vi "Test PA on multiple channels.vi"(11 "Test Case In":refnum<class "NI9375 DI Cont CFG.lvclass">) -> (0 "error out":errorcluster, 3 "Test Case Out":refnum<class "NI9375 DI Cont CFG.lvclass">)   [LabVIEW 2024, in "NI9375 DI Cont CFG.lvclass"]
uses:
  NI9375 DI Cont CFG.lvclass
  NI9375 DI Cont CFG.lvclass/NI9375 DI Cont CFG.ctl
  HAL/MSS/MSS.lvclass
  <vilib>/Astemes/LUnit/Test Case.lvclass
  <vilib>/platform/TimedLoop/XDataNode/XDataNode.xnode
  <vilib>/Platform/TimedLoop/XDataNode/nitl_modes.ctl
  <vilib>/Platform/TimedLoop/XDataNode/XDNodeRunTimeDep.lvlib
  <vilib>/Platform/TimedLoop/XDataNode/wakeup.ctl
  <vilib>/Platform/TimedLoop/XDataNode/timing_clust.ctl
panel:
  out "Error":errorcluster
  in  "stop":bool
  out "Output":variant
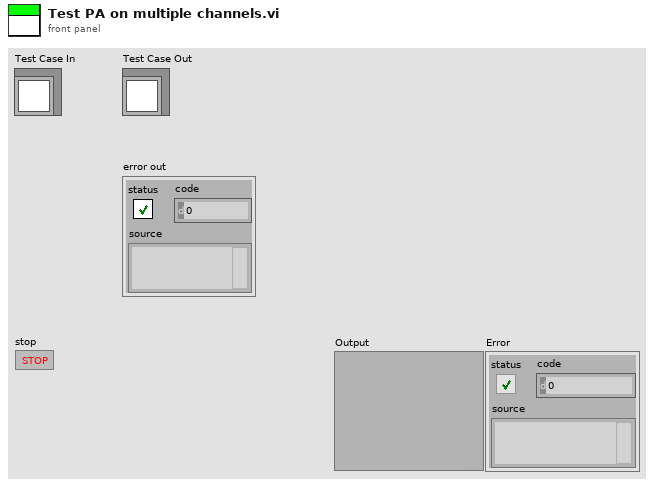
[diagram p1: front panel]
types:
  T1 = typedef "XDNodeRunTimeDep.lvlib/timing_clust.ctl" = cluster{"Expected End [f-1]":u64, "Actual End [f-1]":u64, "Finished Late? [f-1]":bool, "Expected End [i-1]":u64, "Actual End [i-1]":u64, "Finished Late? [i-1]":bool, "Expected Start [i]":u64, "Actual Start [i]":u64, "Expected Start [f]":u64, "Actual Start [f]":u64, "Source Name":string, "Structure Name":string, "Period":i64, "Deadline":i64, "Offset":i64, "Start":i64, "Priority":i32, "Timeout":i32, "Mode":T2, "Wakeup Reason":T3, "Error":errorcluster, "Source Type":string, "Secondary Source Type":string, "Global End Time":u64, "Global Start Time":u64, "Frame Duration":u64, "Iteration Duration":u64, "Assigned CPU":i32, "I/O Scan Engine Mode":u32}
  T2 = typedef "XDNodeRunTimeDep.lvlib/nitl_modes.ctl" = enum32{"No Change", "Process missed periods, maintain original phase", "Discard missed periods, maintain original phase", "Process missed periods, ignore original phase", "Discard missed periods, ignore original phase"}
  T3 = typedef "XDNodeRunTimeDep.lvlib/wakeup.ctl" = enum32{"Normal", "Aborted", "Asynchronous wakeup", "Timing source error", "Timed loop error", "Timeout"}
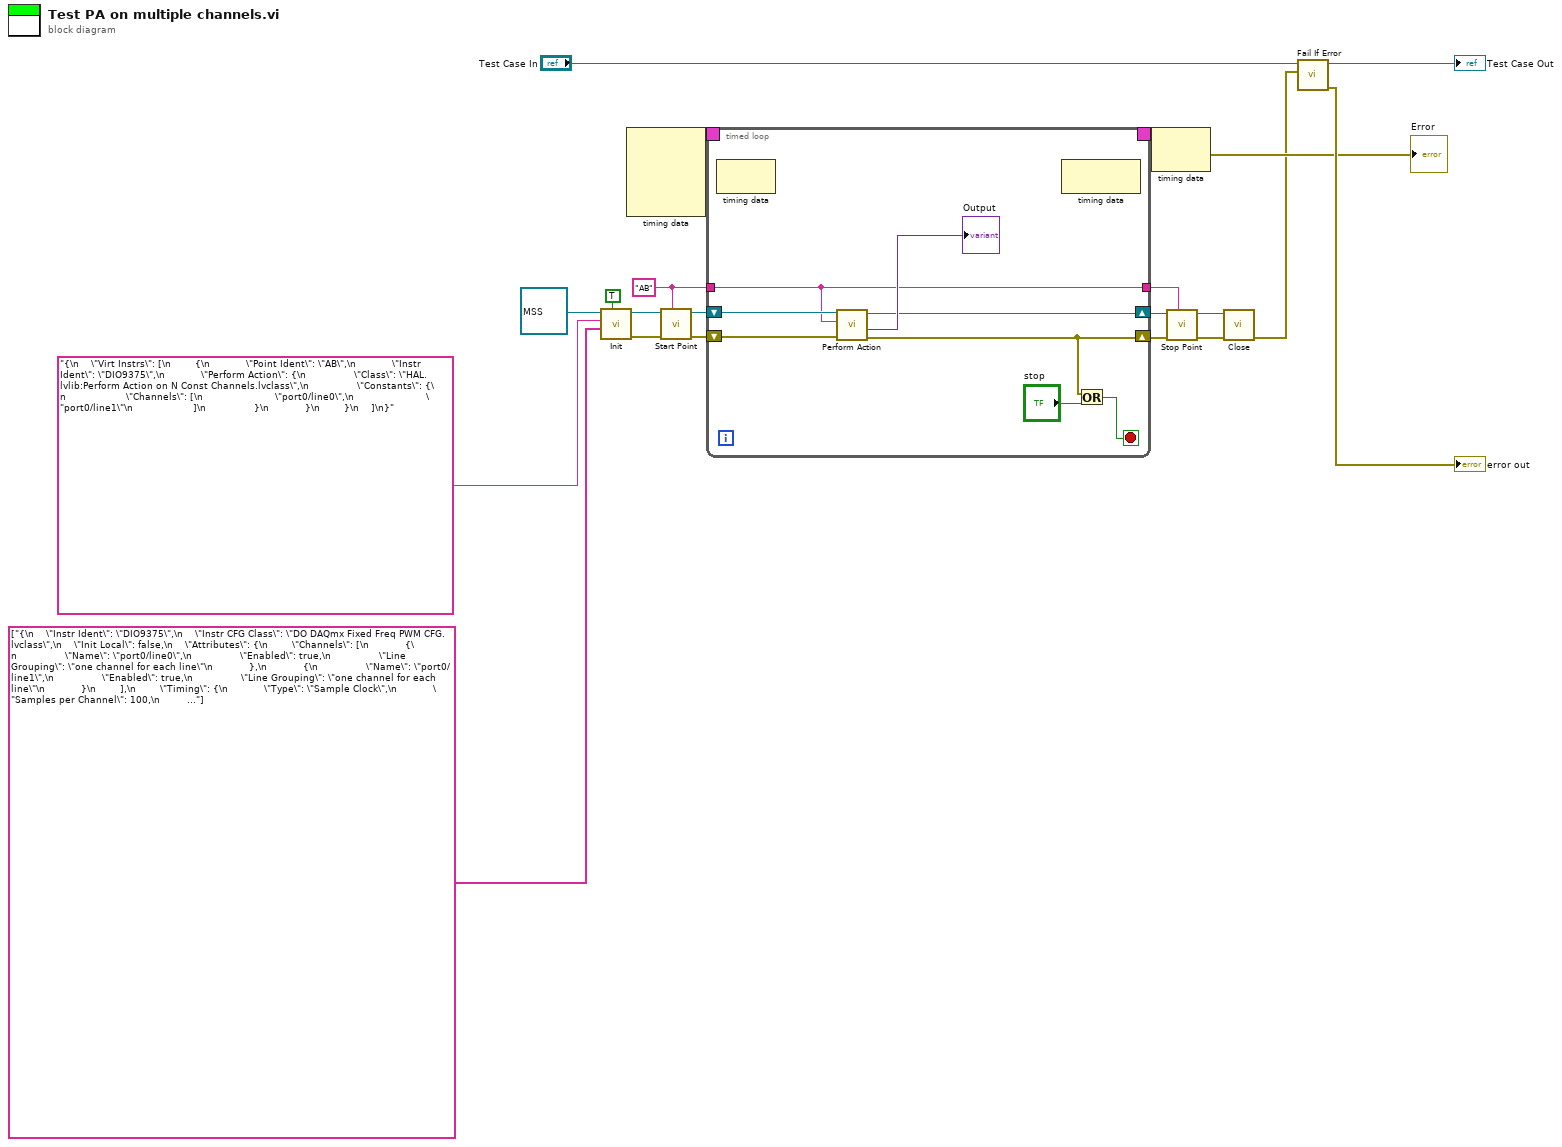
[diagram p0: block diagram]
diagram:
  w9 = "AB" ("Task-Point Ident")
  n1 = call "Init.vi"("Is Target?"=TRUE, "Instr CFGs"=string[] ["{\n    \"Instr Ident\": \"DIO9375\",\n    \"Instr CFG Class\": \"DO DAQmx Fixed Freq PWM CFG.lvclass\",\n    \"Init Local\": false,\n    \"Attributes\": {\n        \"Channels\": [\n            {\n                \"Name\": \"port0/line0\",\n                \"Enabled\": true,\n                \"Line Grouping\": \"one channel for each line\"\n            },\n            {\n                \"Name\": \"port0/line1\",\n                \"Enabled\": true,\n                \"Line Grouping\": \"one channel for each line\"\n            }\n        ],\n        \"Timing\": {\n            \"Type\": \"Sample Clock\",\n            \"Samples per Channel\": 100,\n            \"Sample Mode\": \"Continuous Samples\",\n            \"Sample Rate\": 11,\n            \"Sample Clock Source\": \"OnboardClock\",\n            \"Active Edge\": \"Rising\"\n        },\n        \"Trigger\": {\n            \"Trigger Type\": \"No Trigger\"\n        },\n        \"Generation\": {\n            \"Regen Mode\": \"Allow Regeneration\"\n        }\n    }\n}"], "<JSON> Virt Instr CFG"="{\n    \"Virt Instrs\": [\n        {\n            \"Point Ident\": \"AB\",\n            \"Instr Ident\": \"DIO9375\",\n            \"Perform Action\": {\n                \"Class\": \"HAL.lvlib:Perform Action on N Const Channels.lvclass\",\n                \"Constants\": {\n                    \"Channels\": [\n                        \"port0/line0\",\n                        \"port0/line1\"\n                    ]\n                }\n            }\n        }\n    ]\n}", "MSS in"=refnum<class "MSS.lvclass"> refnum ("HAL.lvlib:MSS.lvclass")) -> ("error out"=w15:errorcluster, "MSS out"=w14:refnum<class "MSS.lvclass">)  [unwired: 4 in, 2 out]
  n2 = node-c288() -> (w11:T1)  [unwired: 4 in]
  n3 = call "Start Point.vi"("Task-Point Ident"=w9, "error in"=w15, "MSS in"=w14) -> ("error out"=w12:errorcluster, "MSS out"=w13:refnum<class "MSS.lvclass">)  [unwired: 7 in]
  n4 = timed-loop {
    timing: w11 -> [_]
    timing-out: [_] -> w10
    tunnel: w9 -> [w25]
    shift-right: [w22] -> w8
    shift-left: w12 -> [w28]
    tunnel: [w25] -> w4
    shift-right: [w24] -> w3
    shift-left: w13 -> [w29]
    stop <- w23 stop-if-true
    n5 = node-c288() -> ()  [unwired: 1 in, 1 out]
    n6 = call "Perform Action.vi"("error in"=w28, "Point Ident"=w25, "MSS in"=w29) -> ("error out"=w22:errorcluster, "Output"=→"Output":variant, "MSS out"=w24:refnum<class "MSS.lvclass">)  [unwired: 5 in, 1 out]
    n7 = node-c288() -> ()  [unwired: 1 in, 1 out]
    n8 = Or(x=w22, y="stop") -> (x .or. y?=w23:bool)
  }
  n9 = node-c288(w10) -> (→"Error":errorcluster)
  n10 = call "Stop Point.vi"("Task-Point Ident"=w4, "error in"=w8, "MSS in"=w3) -> ("error out"=w5:errorcluster, "MSS out"=w1:refnum<class "MSS.lvclass">)  [unwired: 7 in]
  n11 = call "Close.vi"("error in"=w5, "MSS in"=w1) -> ("error out"=w2:errorcluster)  [unwired: 8 in, 1 out]
  n12 = call <vilib>:"Fail If Error.vi"("Assert error"=w2, "LUnit Test Case In"="Test Case In") -> ("error out"=→"error out":errorcluster, "LUnit Test Case Out"=→"Test Case Out":refnum<class "NI9375 DI Cont CFG.lvclass">)  [unwired: 8 in]
